vi "RunPythonFindProbs.vi"(6 "NumIons":bool, 7 "Prob graph ref":refnum<vi>, 9 "Compiler Settings":T1={"Python Path"=path "", "Main File"="mainscript.py", "Meta File"="metascript.txt", "Aux File"="auxscript.py", "Pre File"="metascript.txt"}, 10 "save":i32=1, 11 "filepath":string) -> (2 "standard error":string, 3 "standard output":string)   [LabVIEW 2019]
uses:
  PulseCompiler/CompilerSettings.ctl
panel:
  out "appended array":dbl[][](array[numeric])
  in  "error in (no error)":errorcluster
  out "error out":errorcluster
  out "return code":i32
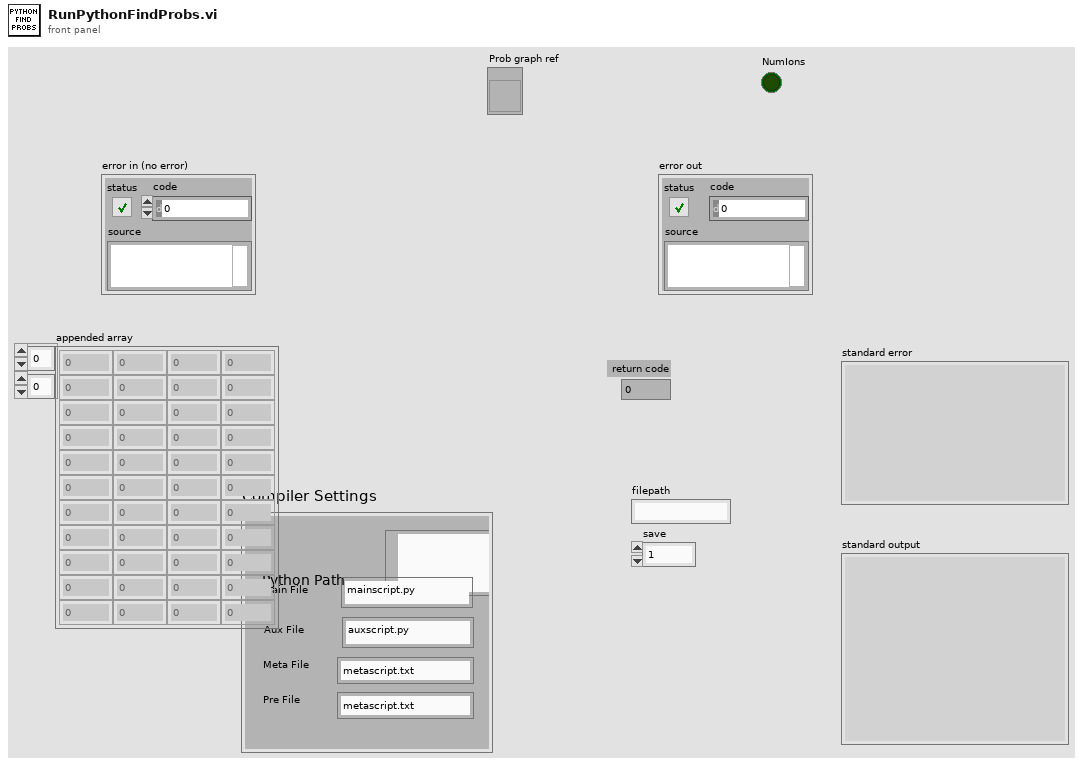
[diagram p1: front panel]
types:
  T1 = typedef "CompilerSettings.ctl" = cluster{"Python Path":path, "Main File":string, "Meta File":string, "Aux File":string, "Pre File":string}
  T2 = cluster{"filepath":string, "save":i32, "num_ions":i32}
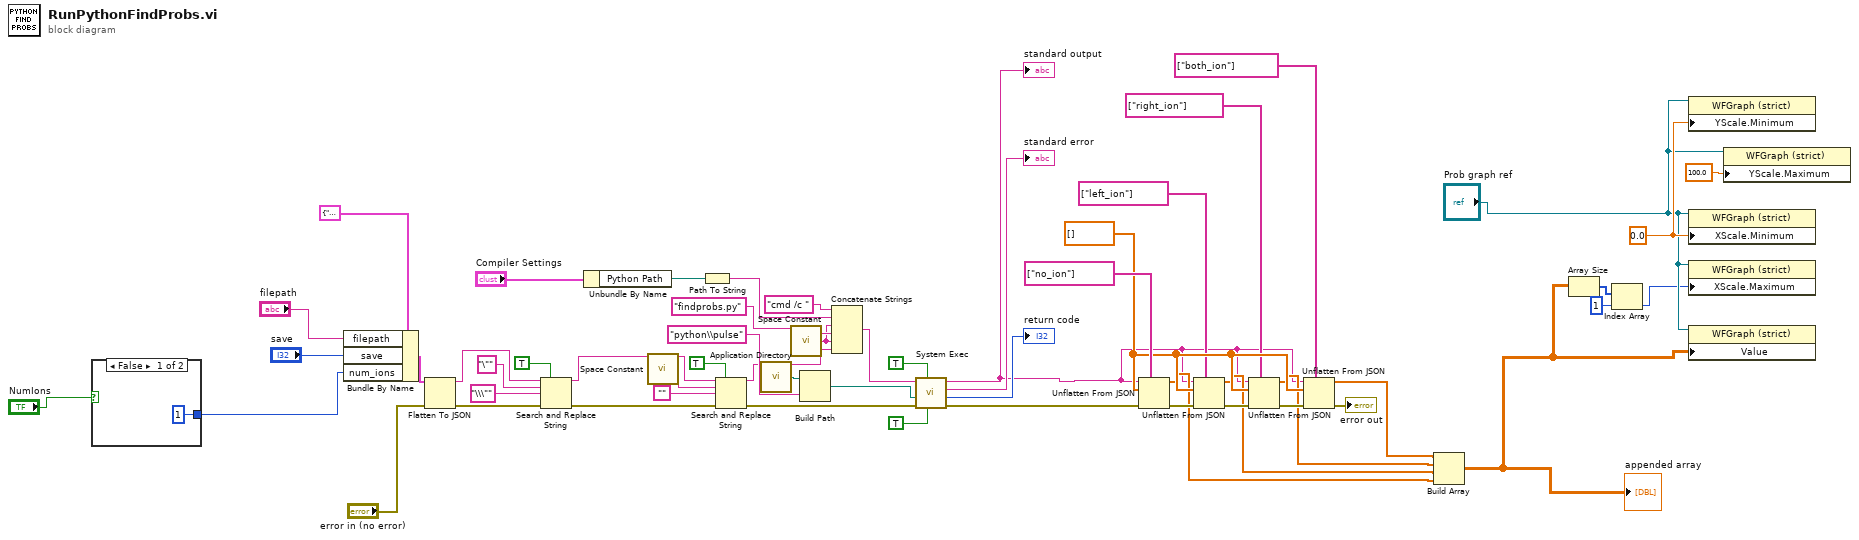
[diagram p0: block diagram]
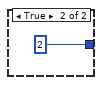
[diagram p2: hidden frame]
diagram:
  w21 = dbl[] []
  w28 = 0.0 ("X Scale.Range:Minimum")
  n1 = case shown="False" "NumIons" {
    tunnel: [1 2] -> w2
    frame False {
    }
    frame True {
    }
  }
  n2 = Bundle By Name(cluster=T2 {"filepath"="", "save"=0, "num_ions"=0}, "filepath"="filepath", "save"="save", "num_ions"=w2) -> (w29:T2)
  n3 = Flatten To JSON(anything=w29, error in (no error)="error in (no error)") -> (JSON string=w42:string, 11:w41:errorcluster)  [unwired: 1 in]
  n4 = Search and Replace String(replace all?=TRUE ("replace all? (F)"), input string=w42, search string="\"", replace string="\\\"" ("replace string (\"\")"), error in=w41) -> (result string=w38:string, error out=w37:errorcluster)  [unwired: 3 in, 2 out]
  n5 = Unbundle By Name("Compiler Settings") -> ("Python Path"=w26:path)
  n6 = call <vilib>:"Space Constant.vi"() -> ("String"=w36:string)
  n7 = Path To String(path=w26) -> (string=w25:string)
  n8 = Search and Replace String(replace all?=TRUE ("replace all? (F)"), input string=w38, search string=w36, replace string="", error in=w37) -> (result string=w34:string, error out=w33:errorcluster)  [unwired: 3 in, 2 out]
  n9 = call <vilib>:"Application Directory.vi"() -> ("Application Directory"=w46:path)
  n10 = call <vilib>:"Space Constant.vi"() -> ("String"=w43:string)
  n11 = Build Path(base path=w46, name or relative path="python\\pulse") -> (appended path=w48:path)
  n12 = Concatenate Strings("cmd /c " ("string"), w25, w43, "findprobs.py" ("name or relative path"), w43, w34) -> (w45:string)
  n13 = call <vilib>:"System Exec.vi"("run minimized? (F)"=TRUE, "wait until completion? (T)"=TRUE, "error in (no error)"=w33, "working directory"=w48, "command line"=w45) -> ("error out"=w8:errorcluster, "return code"=→"return code":i32, "standard error"=→"standard error":string, "standard output"=w9:string)  [unwired: 3 in]
  "standard output" <- w9
  n14 = Unflatten From JSON(path=string[] ["no_ion"], JSON string=w9, type and defaults=w21, error in (no error)=w8) -> (value=w11:dbl[], error out=w17:errorcluster)  [unwired: 3 in]
  n15 = Unflatten From JSON(path=string[] ["left_ion"], JSON string=w9, type and defaults=w21, error in (no error)=w17) -> (value=w10:dbl[], error out=w16:errorcluster)  [unwired: 3 in]
  n16 = Unflatten From JSON(path=string[] ["right_ion"], JSON string=w9, type and defaults=w21, error in (no error)=w16) -> (value=w12:dbl[], error out=w15:errorcluster)  [unwired: 3 in]
  n17 = Unflatten From JSON(path=string[] ["both_ion"], JSON string=w9, type and defaults=w21, error in (no error)=w15) -> (value=w13:dbl[], error out=→"error out":errorcluster)  [unwired: 3 in]
  n18 = Build Array(w13, w12, w10, w11) -> (w6:dbl[][])
  "appended array" <- w6
  n19 = Array Size(array=w6) -> (size(s)=w5:i32[])
  n20 = Index Array(array=w5, index=1) -> (element=w4:i32)
  n21 = property class="WFGraph (strict)"(reference="Prob graph ref", "YScale.Minimum"=w28) -> ()  [unwired: 1 in, 2 out]
  n22 = property class="WFGraph (strict)"(reference="Prob graph ref", "XScale.Minimum"=w28) -> ()  [unwired: 1 in, 2 out]
  n23 = property class="WFGraph (strict)"(reference="Prob graph ref", "XScale.Maximum"=w4) -> ()  [unwired: 1 in, 2 out]
  n24 = property class="WFGraph (strict)"(reference="Prob graph ref", "Value"=w6) -> ()  [unwired: 1 in, 2 out]
  n25 = property class="WFGraph (strict)"(reference="Prob graph ref", "YScale.Maximum"=100.0 ("Y Scale.Range:Maximum")) -> ()  [unwired: 1 in, 2 out]
